vi "Reset Output Protection.vi"(8 "error in (no error)":errorcluster, 11 "VISA resource name":refnum<visa-resource-name>) -> (0 "error out":errorcluster, 3 "VISA resource name out":refnum<visa-resource-name>)   [LabVIEW 2020, in "RIGOL DP1000 Series.lvlib"]
doc: "Resets the status of over voltage protection (OVP) and over current protection (OCP)."
uses:
  <instrlib>/RIGOL DP1000 Series/RIGOL DP1000 Series.lvlib
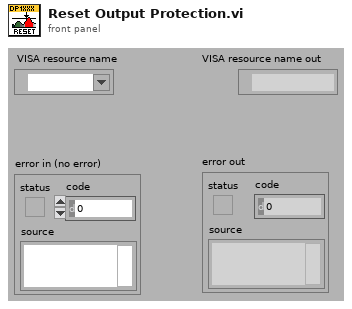
[diagram p1: front panel]
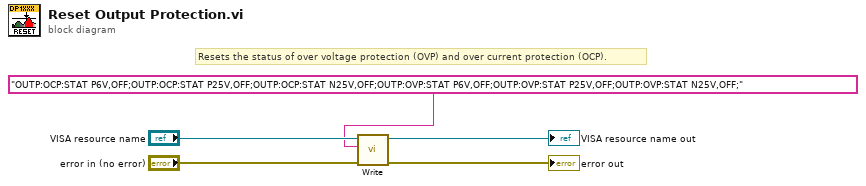
[diagram p0: block diagram]
diagram:
  # "Resets the status of over voltage protection (OVP) and over current protection (OCP)."
  n1 = call <instrlib>:"Write.vi"("error in (no error)"="error in (no error)", "Write Buffer (\"\")"="OUTP:OCP:STAT P6V,OFF;OUTP:OCP:STAT P25V,OFF;OUTP:OCP:STAT N25V,OFF;OUTP:OVP:STAT P6V,OFF;OUTP:OVP:STAT P25V,OFF;OUTP:OVP:STAT N25V,OFF;", "VISA resource name"="VISA resource name") -> ("error out"=→"error out":errorcluster, "VISA resource name out"=→"VISA resource name out":refnum<visa-resource-name>)  [unwired: 7 in]
